vi "RTS Create Listbox Data.vi"(11 "Full List Box Data":string[][](array[string])) -> (1 "Custom Titles":string[](array[string]), 3 "Custom Listbox Data":string[][](array[string]), 5 "Point File Name":string)   [LabVIEW 2020]
uses:
  Type Definitions/RTS Point File.ctl
panel:
  out "path":path
  out "Point File":T1[](array[typedef])
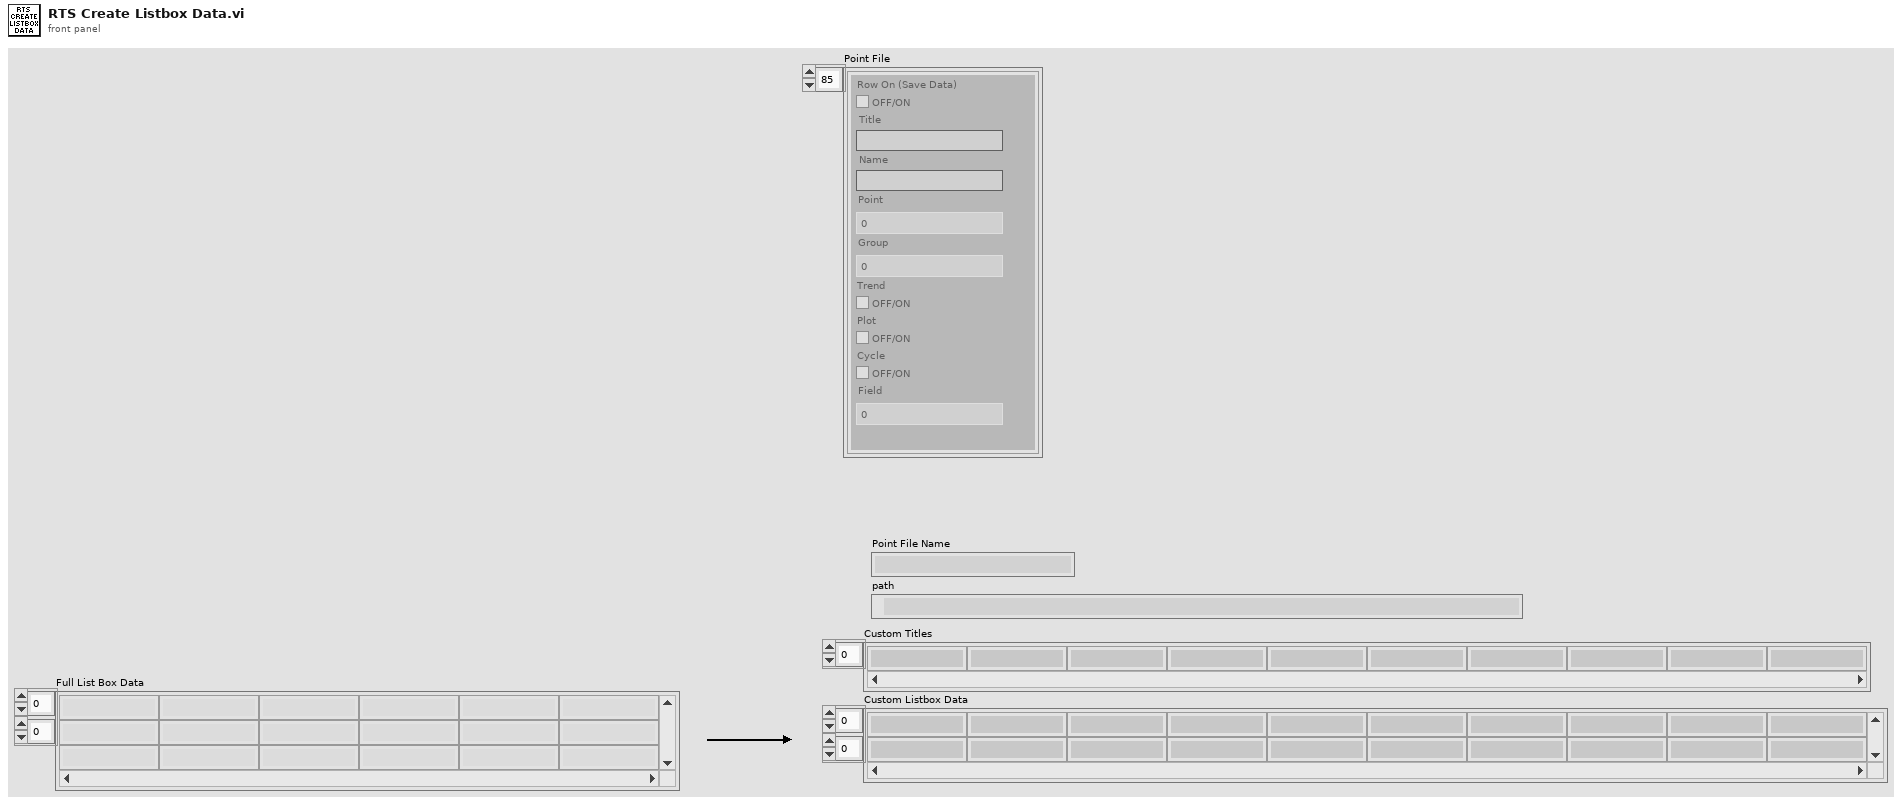
[diagram p1: front panel]
types:
  T1 = typedef "RTS Point File.ctl" = cluster{"Title":string, "Name":string, "Point":u8, "Plot":bool, "Trend":bool, "Cycle":bool, "Field":u8, "Row On (Save Data)":bool, "Group":u8}
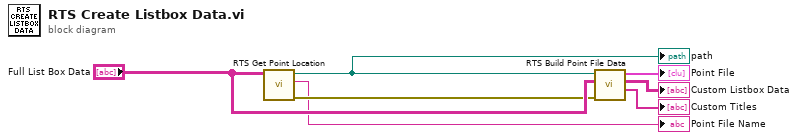
[diagram p0: block diagram]
diagram:
  n1 = call "RTS Get Point Location.vi"("Full List Box Data"="Full List Box Data") -> ("Error Out"=w2:errorcluster, "Point File Name"=→"Point File Name":string, "Path"=w3:path)  [unwired: 8 in]
  "path" <- w3
  n2 = call "RTS Build Point File Data.vi"("Error In"=w2, "Full List Box Data"="Full List Box Data", "Point File Location"=w3) -> ("Custom Titles"=→"Custom Titles":string[], "Custom Listbox Data"=→"Custom Listbox Data":string[][], "Point File"=→"Point File":T1[])  [unwired: 5 in, 1 out]
